vi "Levelmeter_He_readout.vi"(11 "stop DAQ":bool) -> (1 "He-Pot in (%)":dbl, 2 "He Bath (%)":dbl)   [LabVIEW 2019]
uses:
  Global/Global Variables/Data_Display_global.vi
  <vilib>/ptbypt/NI_PtbyPt.lvlib
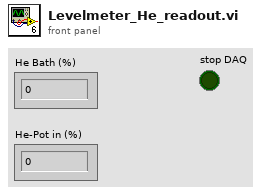
[diagram p1: front panel]
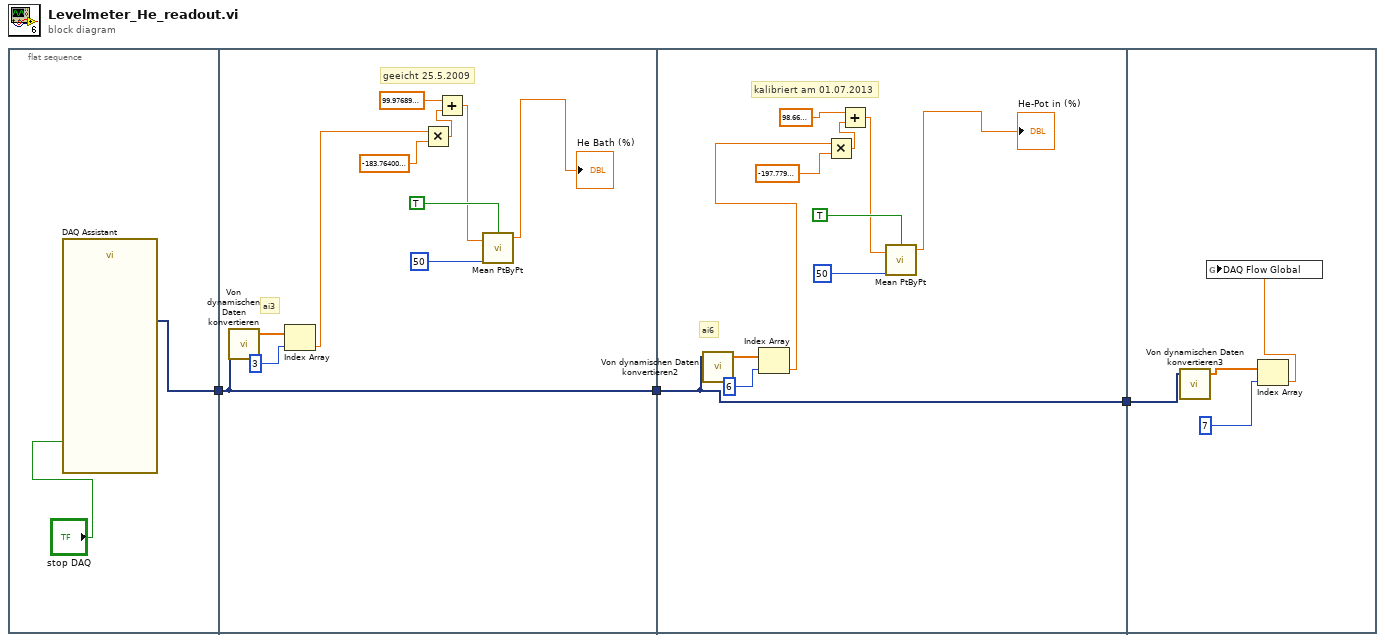
[diagram p0: block diagram]
diagram:
  n1 = flat-sequence {
    tunnel: [w5] -> w3
    tunnel: w3 -> [w14]
    tunnel: [w14] -> w2
    tunnel: w2 -> [w17]
    tunnel: [w17] -> w1
    tunnel: w1 -> [w29]
    frame #0 {
      n2 = call "DAQ Assistant"("stop (T)"="stop DAQ") -> ("data"=w5:dynamicdata)  [unwired: 16 in, 2 out]
    }
    frame #1 {
      # "geeicht 25.5.2009"
      # "ai3"
      n3 = call "Von dynamischen Daten konvertieren"("Dynamic Data Type"=w14) -> ("Array"=w16:dbl[])  [unwired: 3 in]
      n4 = Index Array(array=w16, index=3) -> (element=w7:dbl)
      n5 = Multiply(x=w7, y=sgl -183.764 ("x")) -> (x*y=w12:dbl)
      n6 = Add(x=sgl 99.9769, y=w12) -> (x+y=w8:dbl)
      n7 = call <vilib>:"Mean PtByPt.vi"("x"=w8, "sample length"=50 ("index"), "initialize"=TRUE) -> ("mean"=→"He Bath (%)":dbl)  [unwired: 1 in, 1 out]
    }
    frame #2 {
      # "kalibriert am 01.07.2013"
      # "ai6"
      n8 = call "Von dynamischen Daten konvertieren2"("Dynamic Data Type"=w17) -> ("Array"=w27:dbl[])  [unwired: 3 in]
      n9 = Index Array(array=w27, index=6) -> (element=w19:dbl)
      n10 = Multiply(x=w19, y=sgl -197.78 ("x")) -> (x*y=w25:dbl)
      n11 = Add(x=sgl 98.66, y=w25) -> (x+y=w22:dbl)
      n12 = call <vilib>:"Mean PtByPt.vi"("x"=w22, "sample length"=50 ("index"), "initialize"=TRUE) -> ("mean"=→"He-Pot in (%)":dbl)  [unwired: 1 in, 1 out]
    }
    frame #3 {
      n13 = call "Von dynamischen Daten konvertieren3"("Dynamic Data Type"=w29) -> ("Array"=w30:dbl[])  [unwired: 3 in]
      n14 = Index Array(array=w30, index=7) -> (element=w28:dbl)
      n15 = global write "Data_Display_global.vi" "DAQ Flow Global"(w28) -> ()
    }
  }
